vi "Auto_RangeStatus.vi"(0 "VisaCluster":T1, 11 "error in (no error)":errorcluster) -> (4 "VisaCluster":T1, 6 "Display":string, 8 "Answer":string, 10 "Auto_Range":bool, 15 "error out":errorcluster)   [LabVIEW 2014, in "FH 55.lvlib"]
doc: "Diese VI zeigt ob die Auto-Taste führ die automatische Messbereichswahl eingeschaltet oder ausgeschaltet ist.\n\nThis VI shows that the Auto-keys perform the automatic range selection is switched on or off."
uses:
  FH 55.lvlib
  TypeDef/VisaCluster.ctl
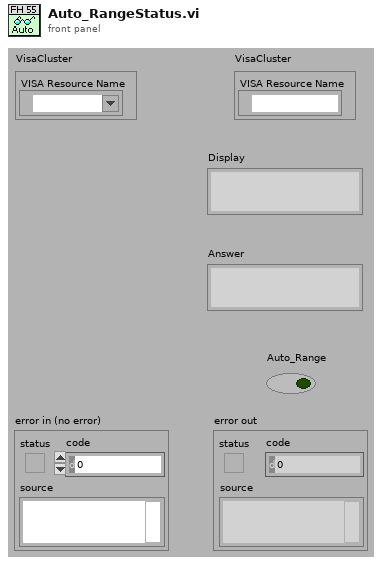
[diagram p1: front panel]
types:
  T1 = typedef "FH 55.lvlib/VisaCluster.ctl" = cluster{"VISA Resource Name":refnum<visa-resource-name>}
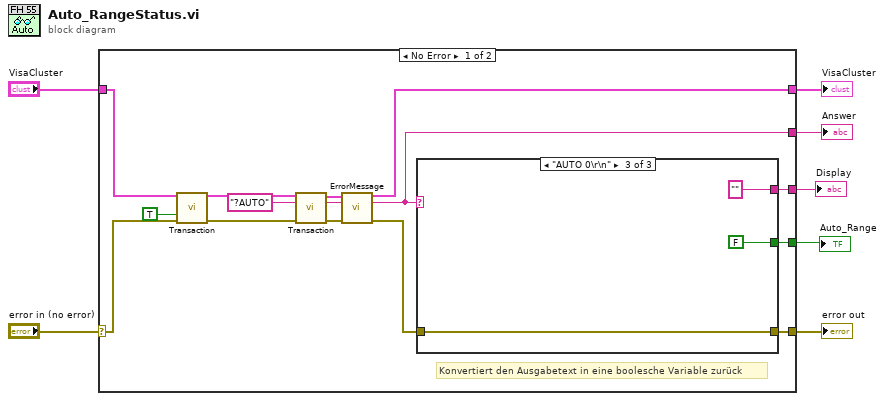
[diagram p0: block diagram]
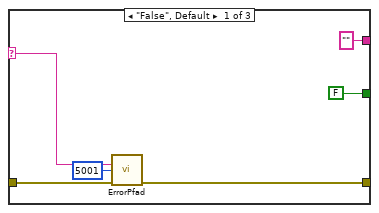
[diagram p2: hidden frame]
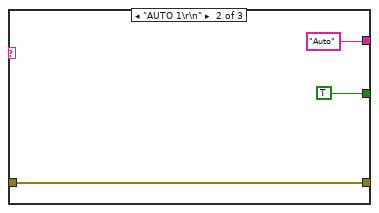
[diagram p3: hidden frame]
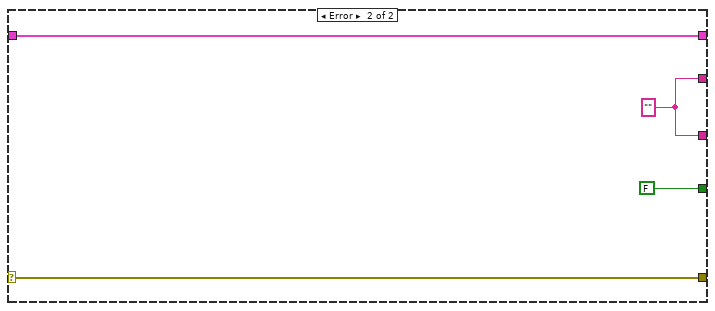
[diagram p4: hidden frame]
diagram:
  n1 = case shown="No Error" "error in (no error)" {
    selector: "error in (no error)" -> [w18 w37]
    tunnel: "VisaCluster" -> [w16 w38]
    tunnel: [w22 w38] -> w3
    tunnel: [w11 w37] -> w5
    tunnel: [w9 w35] -> w4
    tunnel: [w13 FALSE] -> w2
    tunnel: [w8 w35] -> w1
    frame No Error {
      # "Konvertiert den Ausgabetext in eine boolesche Variable zurück"
      n2 = call "Transaction.vi"("VisaCluster"=w16, "Read Only? (False)"=TRUE, "error in (no error)"=w18) -> ("VisaCluster"=w15:T1, "error out"=w17:errorcluster)  [unwired: 9 in, 2 out]
      n3 = call "Transaction.vi"("VisaCluster"=w15, "Command"="?AUTO", "error in (no error)"=w17) -> ("VisaCluster"=w20:T1, "Answer"=w10:string, "error out"=w21:errorcluster)  [unwired: 9 in, 1 out]
      n4 = call "ErrorMessage.vi"("VisaCluster"=w20, "Message In"=w10, "error in (no error)"=w21) -> ("VisaCluster"=w22:T1, "Message Out"=w9:string, "error out"=w12:errorcluster)  [unwired: 10 in]
      n5 = case shown="\"AUTO 0\\r\\n\"" w9 {
        selector: w9 -> [w24 _ _]
        tunnel: [FALSE TRUE FALSE] -> w13
        tunnel: w12 -> [w27 w30 w33]
        tunnel: [w26 w30 w33] -> w11
        tunnel: ["" "Auto" ""] -> w8
        frame "False", Default {
          n6 = call "ErrorPfad.vi"("Message In"=w24, "Numeric"=5001, "error in (no error)"=w27) -> ("error out"=w26:errorcluster)  [unwired: 11 in, 1 out]
        }
        frame "AUTO 1\r\n" {
        }
        frame "AUTO 0\r\n" {
        }
      }
    }
    frame Error {
      w35 = ""
    }
  }
  "error out" <- w5
  "Answer" <- w4
  "VisaCluster" <- w3
  "Auto_Range" <- w2
  "Display" <- w1
